vi "createRecord.Error.vi"(6 "Serializer":refnum<class "Serializer.lvclass">, 7 "Level":T1(ring), 8 "error in (no error)":errorcluster, 9 "Error":errorcluster, 10 "Message":string, 11 "Record.Error in":refnum<class "Record.Error.lvclass">) -> (0 "error out":errorcluster, 3 "Record.Error out":refnum<class "Record.Error.lvclass">)   [LabVIEW 2017, in "Error Log.lvlib" / "Record.Error.lvclass"]
uses:
  Record.Error.lvclass
  \\192.168.1.40\Neosoft/Partage/Dossiers Personnels/BRO/DevTools_BR/wc/ErrorLog/src/Record/Record.lvclass
  Serializer/Serializer.lvclass
  Record.Error.lvclass/Record.Error.ctl
  Record/Record.lvclass
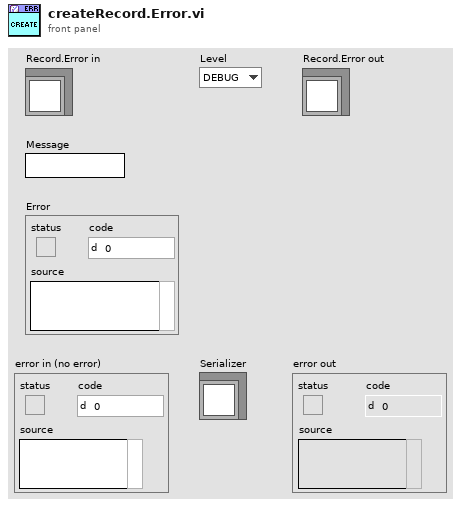
[diagram p1: front panel]
types:
  T1 = enum16{"DEBUG", "INFO", "WARNING", "ERROR", "CRITICAL"}
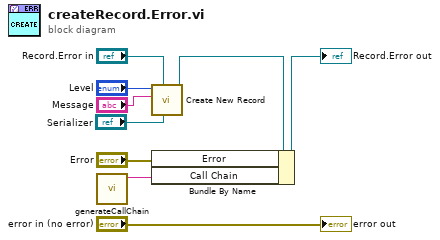
[diagram p0: block diagram]
diagram:
  n1 = call "generateCallChain.vi"() -> ("Callchain"=w6:string)  [unwired: 11 in]
  n2 = call "Create New Record.vi"("Serializer"="Serializer", "Record in"="Record.Error in", "Message"="Message", "Level"="Level") -> ("Record out"=w4:refnum<class "Record.Error.lvclass">)  [unwired: 6 in, 1 out]
  n3 = Bundle By Name(cluster=w4, "Error"="Error", "Call Chain"=w6) -> (→"Record.Error out":refnum<class "Record.Error.lvclass">)
  "error out" <- "error in (no error)"
